vi "Waveform simulator.vi"(9 "Waveform Parameters":T1, 10 "Digitizing Parameters":T2) -> (2 "Waveform Output":cluster{"time":dbl[], "displacement":dbl[]})   [LabVIEW 2015]
uses:
  <vilib>/imath/engines/lvmath2/RunTimeEngine/Managers/WorkSpace/UID Generator.vi
  <vilib>/imath/engines/lvmath2/RunTimeEngine/RunTimeType/NIMS_RunTimeType_From StrictType (excl LVString).vi
  <instcachedir>/0/NIMS_RunTimeType_From StrictType (excl LVString)_EB1C38A9BC5048DA9ABDA8F781E54D21.lvgen/NIMS_RunTimeType_From StrictType (excl LVString)_EB1C38A9BC5048DA9ABDA8F781E54D21_000.vi
  <vilib>/imath/engines/lvmath2/RunTimeEngine/LocalVariableDefStatement/MC_LocalVariableDefStatement_Display.vi
  <vilib>/imath/engines/lvmath2/RunTimeEngine/RangeToken/NIMS_Range.vi
  <instcachedir>/0/NIMS_Range_D919CC09935940E88F755EC1C6F49AC1.lvgen/NIMS_Range_D919CC09935940E88F755EC1C6F49AC1_000.vi
  <vilib>/imathl/engines/lvmath/Functions/Error Handling/Create Error.vi
  <vilib>/imath/engines/lvmath2/RunTimeEngine/ArithmeticOperatorToken/NIMS_ArithmeticOperator_times.vi
  <instcachedir>/0/NIMS_ArithmeticOperator_times_DF26C4080E2A467BA28C929B8CF31953.lvgen/NIMS_ArithmeticOperator_times_DF26C4080E2A467BA28C929B8CF31953_000.vi
  <vilib>/imath/engines/lvmath2/RunTimeEngine/Managers/SymbolTable/Clear UID.vi
  <vilib>/imath/engines/lvmath2/RunTimeEngine/NodeEndStatement/NIMS_NodeEndStatement_Output.vi
  <instcachedir>/0/NIMS_NodeEndStatement_Output_53EC0D466D134D7ABD903AC30B43404B.lvgen/NIMS_NodeEndStatement_Output_53EC0D466D134D7ABD903AC30B43404B_005.vi
  <vilib>/imath/engines/lvmath2/RunTimeEngine/ErrorHandling/NIMS_Finalize Error.vi
  <vilib>/imath/engines/lvmath2/RunTimeEngine/Managers/SymbolTable/NIMS_WorkSpace.lvlib
panel:
  out "XY Graph":cluster{"t":dbl[], "x":dbl[]}(graph)
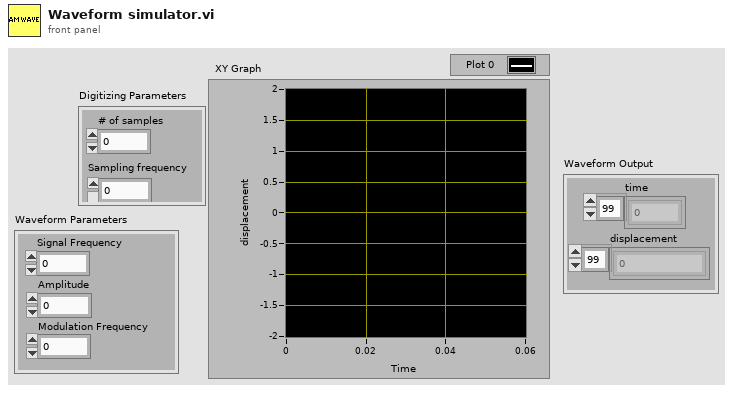
[diagram p1: front panel]
types:
  T1 = cluster{"Signal Frequency":dbl, "Amplitude":dbl, "Modulation Frequency":dbl}
  T2 = cluster{"# of samples":dbl, "Sampling frequency":dbl}
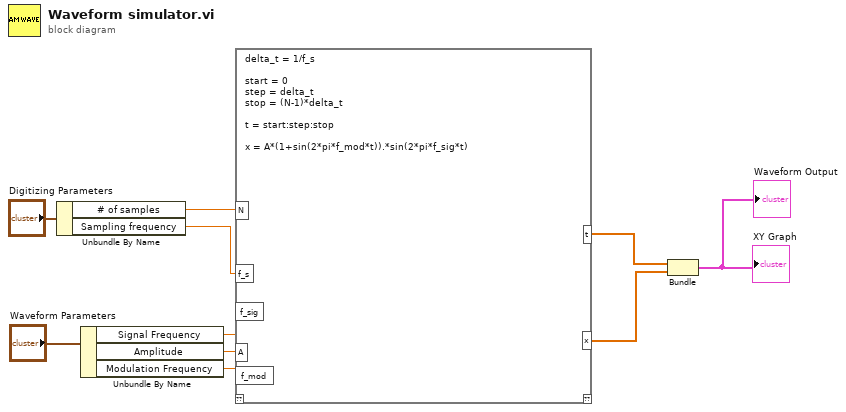
[diagram p0: block diagram]
diagram:
  n1 = Unbundle By Name("Digitizing Parameters") -> ("# of samples"=w7:dbl, "Sampling frequency"=w6:dbl)
  n2 = Unbundle By Name("Waveform Parameters") -> ("Signal Frequency"=w2:dbl, "Amplitude"=w4:dbl, "Modulation Frequency"=w3:dbl)
  n3 = mathscript code="delta_t = 1/f_s\n\nstart = 0\nstep = delta_t\nstop = (N-1)*delta_t\n\nt = start:step:stop\n\nx = A*(1+sin(2*pi*f_mod*t)).*sin(2*pi*f_sig*t)"("N"=w7, "f_s"=w6, "f_sig"=w2, "A"=w4, "f_mod"=w3) -> ("x"=w9:dbl[], "t"=w10:dbl[])  [unwired: 1 in, 1 out]
  n4 = Bundle("t"=w10, "x"=w9) -> (→"XY Graph" →"Waveform Output":cluster{"t":dbl[], "x":dbl[]})  [unwired: 1 in]
